vi "Init.vi"(8 "Error In":errorcluster, 10 "Colour":u32(colorbox), 11 "Snake In":refnum<class "Snake.lvclass">) -> (0 "Error Out":errorcluster, 3 "object out":refnum<class "Snake.lvclass">)   [LabVIEW 2021, in "Snake.lvclass"]
uses:
  Snake.lvclass
  C:/Users/poche/Programs/LabVIEW/Imposible_Snake/GameEl_class/GameEl.lvclass
  Snake Status.ctl
  GameEl_class/GameEl.lvclass/GameEl.ctl
  Snake.lvclass/Snake.ctl
  GameEl_class/GameEl.lvclass
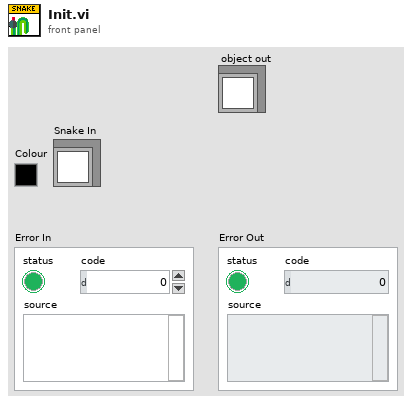
[diagram p1: front panel]
types:
  T1 = typedef "Snake.lvclass/Snake Status.ctl" = cluster{"Boosters":cluster{"Shield":bool, "Star":bool}, "Weakeners":cluster{"Grapes":bool, "Bomb Crash":bool, "Death":bool}}
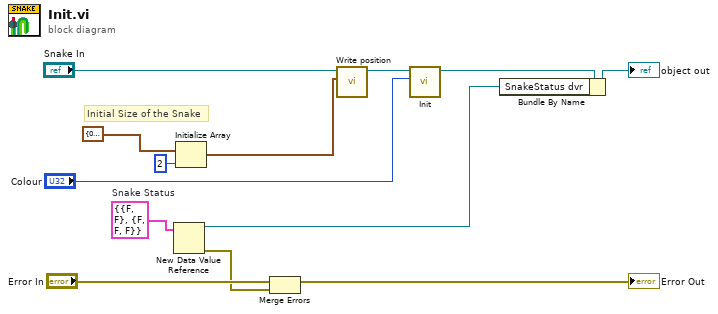
[diagram p0: block diagram]
diagram:
  w9 = T1 {"Boosters"={"Shield"=FALSE, "Star"=FALSE}, "Weakeners"={"Grapes"=FALSE, "Bomb Crash"=FALSE, "Death"=FALSE}}  # Snake Status
  # "Initial Size of the Snake"
  n1 = New Data Value Reference(data value=w9) -> (data value reference=w4:refnum<data-value>, error out=w5:errorcluster)  [unwired: 1 in]
  n2 = Initialize Array(cluster{"x":dbl, "y":dbl} {"x"=0.0, "y"=0.0} ("position"), 2 ("dimension size")) -> (w1:cluster{"x":dbl, "y":dbl}[])
  n3 = Merge Errors("Error In", w5) -> (→"Error Out":errorcluster)
  n4 = call "Write position.vi"("position"=w1, "GameEl in"="Snake In") -> ("GameEl out"=w2:refnum<class "Snake.lvclass">)  [unwired: 8 in, 1 out]
  n5 = call-parent "Init.vi"("Colour"="Colour", "GameEl in"=w2) -> ("GameEl out"=w11:refnum<class "Snake.lvclass">)  [unwired: 8 in, 1 out]
  n6 = Bundle By Name(cluster=w11, "SnakeStatus dvr"=w4) -> (→"object out":refnum<class "Snake.lvclass">)
